vi "Listen for New Connections.vi"(8 "error in (no error)":errorcluster, 11 "State Variables":T1) -> (0 "error out":errorcluster)   [LabVIEW 2015, in "Control Addon Engine.lvlib"]
uses:
  Types/Network Engine State Variables.ctl
  <vilib>/NI/NI VeriStand Inline Async API/_VS Inline Async API/Process/Process.lvclass
  <vilib>/NI/STM/Connection Manager/TCP/Advanced/TCP Connection Manager Reference.ctl
  <vilib>/NI/STM/Connection Manager/TCP/Advanced/TCP Connection Manager State Variables.ctl
  <vilib>/NI/STM/TCP/TCP Connection Info.ctl
  <vilib>/NI/STM/SubVIs/MetaDataElement.ctl
  <vilib>/NI/STM/Connection Manager/TCP/TCP Connection Properties.ctl
  <vilib>/NI/STM/TCP/TCP Read Options.ctl
  <vilib>/NI/STM/Connection Manager/TCP/TCP Connection Method.ctl
  <vilib>/NI/NI VeriStand Inline Async API/_VS Inline Async API/Process/Process.lvclass/Process.ctl
  <vilib>/NI/STM/TCP/Read Meta Data (TCP Ref).vi
  <vilib>/NI/NI VeriStand Inline Async API/_VS Inline Async API/Error Handling Process/SubVIs/Error.ConvertArray.vi
  <vilib>/NI/STM/TCP/Read Meta Data (TCP Clst).vi
  Control Addon Engine.lvlib
  <vilib>/NI Veristand/Custom Device Tools/Custom Device Utility Library/Custom Device Utility Library.lvlib
  <vilib>/NI/STM/NI STM.lvlib
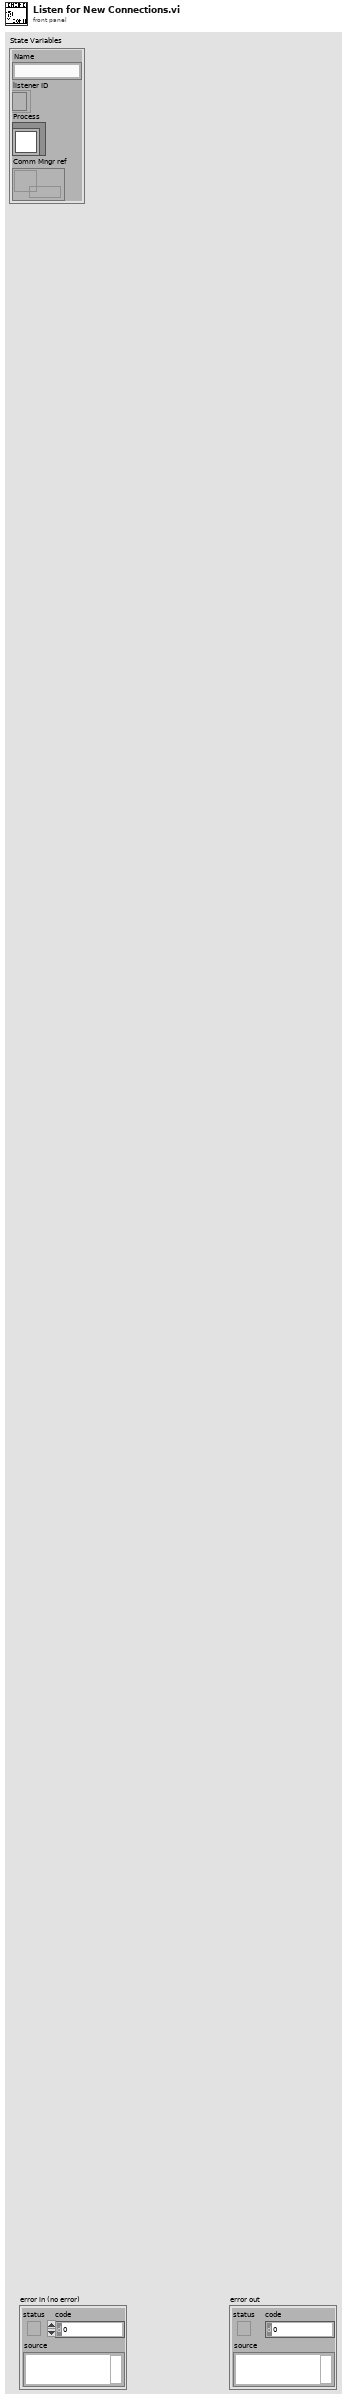
[diagram p1: front panel]
types:
  T1 = typedef "Control Addon Engine.lvlib/Network Engine State Variables.ctl" = cluster{"Name":string, "listener ID":refnum<k5>, "Process":refnum<class "Process.lvclass">, "Comm Mngr ref":T2}
  T2 = typedef "TCP Connection Manager Reference.ctl" = refnum<data-value>
  T3 = typedef "NI STM.lvlib/TCP Read Options.ctl" = cluster{"ignore timeout error":bool, "timeout ms (1000)":i32}
  T4 = typedef "NI STM.lvlib/TCP Connection Method.ctl" = enum16{"Initialize", "Add Connection", "Set Properties", "Get Connection(s)", "Remove Connection", "Remove All Connections", "Get Connection Count"}
  T5 = typedef "NI STM.lvlib/TCP Connection Properties.ctl" = cluster{"Name":string, "Address":string, "Custom":string}
  T6 = typedef "NI STM.lvlib/TCP Connection Info.ctl" = cluster{"connection ID":refnum<k5>, "meta data":T7[]}
  T7 = typedef "NI STM.lvlib/MetaDataElement.ctl" = string
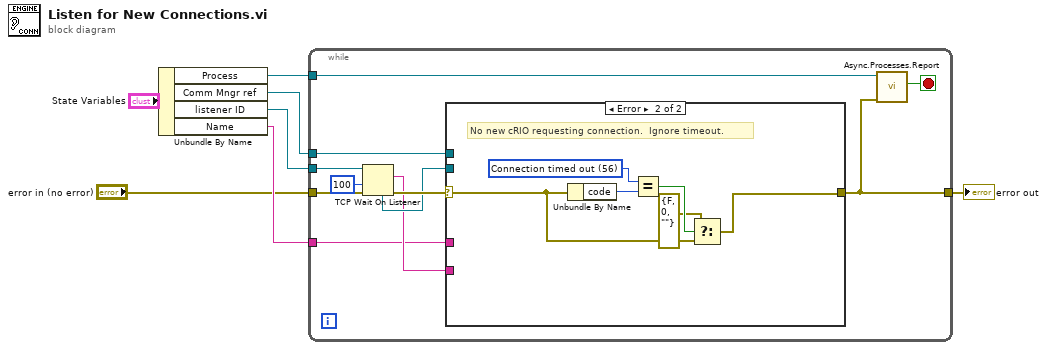
[diagram p0: block diagram]
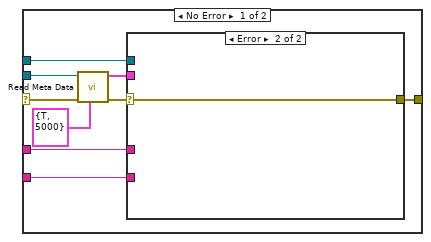
[diagram p2: hidden frame]
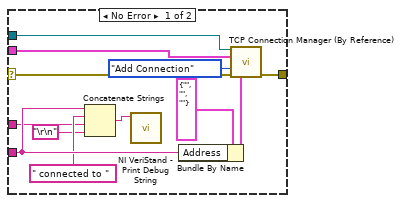
[diagram p3: hidden frame]
diagram:
  n1 = Unbundle By Name("State Variables") -> ("Process"=w6:refnum<class "Process.lvclass">, "Comm Mngr ref"=w5:T2, "listener ID"=w4:refnum<k5>, "Name"=w7:string)
  n2 = while {
    tunnel: "error in (no error)" -> [w18]
    tunnel: w4 -> [w17]
    tunnel: [w9] -> w2
    tunnel: w5 -> [w12]
    tunnel: w7 -> [w11]
    tunnel: w6 -> [w10]
    stop <- w8 stop-if-true
    n3 = TCP Wait On Listener(8:w18, 9:100 ("timeout ms (wait forever: -1)"), 11:w17) -> (0:w15:errorcluster, 2:w13:string, 4:w14:refnum<k5>)  [unwired: 1 in, 2 out]
    n4 = case shown="Error" w15 {
      selector: w15 -> [w27 w43]
      tunnel: w14 -> [w26 _]
      tunnel: [w24 w42] -> w9
      tunnel: w13 -> [w21 _]
      tunnel: w12 -> [w23 _]
      tunnel: w11 -> [w20 _]
      frame No Error {
        n5 = call-poly <vilib>:"Read Meta Data.vi"("options"=T3 {"ignore timeout error"=TRUE, "timeout ms (1000)"=5000}, "error in"=w27, "connection ID"=w26) -> ("error out"=w22:errorcluster, "connection info out"=w25:T6)  [unwired: 6 in, 1 out]
        n6 = case shown="Error" w22 {
          selector: w22 -> [w36 w40]
          tunnel: w21 -> [w34 _]
          tunnel: w25 -> [w39 _]
          tunnel: [w38 w40] -> w24
          tunnel: w23 -> [w37 _]
          tunnel: w20 -> [w32 _]
          frame No Error {
            n7 = Concatenate Strings(w34, " connected to " ("string"), w32, "\r\n") -> (w35:string)
            n8 = call <vilib>:"NI VeriStand - Print Debug String.vi"("Message"=w35) -> ()  [unwired: 10 in, 1 out]
            n9 = Bundle By Name(cluster=T5 {"Name"="", "Address"="", "Custom"=""} ("properties in"), "Address"=w34) -> (w29:T5)
            n10 = call <vilib>:"TCP Connection Manager (By Reference).vi"("connection manager ref in"=w37, "connection in"=w39, "method"=TCP_Connection_Method."Add Connection", "error in"=w36, "properties in"=w29) -> ("error out"=w38:errorcluster)  [unwired: 4 in, 6 out]
          }
          frame Error {
          }
        }
      }
      frame Error {
        w44 = 56 items=["No Error", "Argument Error", "Memory Full", "Out of Zone", "End of File", "File Already Open", "Generic File IO Error", "File Not Found", "File Permission Error", "Disk Full", "Duplicate Path", "Too Many Files Open", "Not Enabled", "Resource File Not Found", "Cannot Add Resource", "Resource Not Found", "Image Not Found", "Image Memory Error", "Pen Does Not Exist", "Config Bad Type", "Config Token Not Found", "Config Parse Error", "Config Memory Error", "Bad External Code Format", "Bad External Code Offset", "External Code Not Present", "Null Window", "Destroy Window Mixup", "Null Menu", "Print Aborted", "Bad Print Record", "Print Driver Error", "Windows Error During Print", "Memory Error During Print", "Print Dialog Error", "Generic Print Error", "Invalid Device Refnum", "Device Not Found", "Device Parameter Error", "Device Unit Error", "Can't Open Device", "Device Call Aborted", "Generic Error", "Cancelled By User", "Object ID Too Low", "Object ID Too High", "Object Not In Heap", "Unknown Heap", "Bad DefProc ID", "DefProc Not In Table", "Message Out Of Range", "Null Method", "Unknown Message", "Manager Call Not Supported", "Bad address", "Connection In progress", "Connection timed out", "Connection is already in progress", "Network attribute not supported", "Network error", "Address in use", "System out of memory", "Connection aborted", "Connection refused", "Connection is not connected", "Connection is already connected", "Connection closed", "Initialize error (interapplication manager)", "Bad occurrence", "Wait on unbound occurrence handler", "Occurrence queue overflow", "Bad path", "Semaphore not signaled", "Unrecognized type (interapplication manager)"] ("1st Error to Convert")
        # "No new cRIO requesting connection.  Ignore timeout."
        n11 = Unbundle By Name(w43) -> ("code"=w45:i32)
        n12 = Equal?(x=w44, y=w45) -> (x = y?=w46:bool)
        n13 = Select(t=errorcluster {"status"=FALSE, "code"=0, "source"=""} ("error in (no error)"), s=w46, f=w43) -> (s? t:f=w42:errorcluster)
      }
    }
    n14 = call <vilib>:"Async.Processes.Report.vi"("Error"=w9, "Process in"=w10) -> ("Stop"=w8:bool)  [unwired: 8 in, 1 out]
  }
  "error out" <- w2
